vi "VCA_S.vi"(6 "EG":fxp<+,8,0>=0.99609375, 8 "Amount":fxp<+,8,0>=0.99609375, 9 "Sample In":fxp<+/-,8,8>) -> (1 "Sample Out":fxp<+/-,8,8>)   [LabVIEW 2015]
doc: "Includes two steps of amplitude control, adding flexibility to more complex signal generator designs.\n\nThe latency of this VI is 14 cycles."
uses:
  <vilib>/rvi/FXPMathLib/FxpMul/XNode/nifxpmath_Multiplier.xnode
  <vilib>/rvi/FXPMathLib/sim/FxpSim.dll
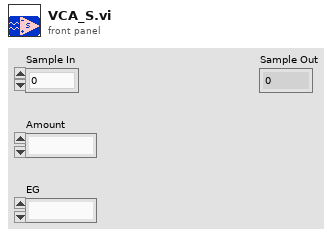
[diagram p1: front panel]
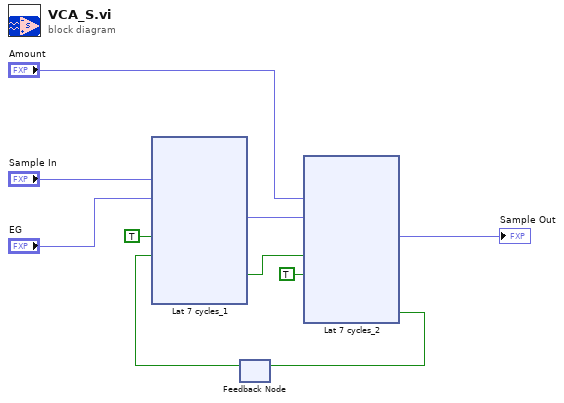
[diagram p0: block diagram]
diagram:
  n1 = feedback #1() -> (w3:bool)  [unwired: 1 in]
  n2 = xnode "Lat 7 cycles_1"("x"="Sample In", "y"="EG", "input valid"=TRUE, "ready for output (T)"=w3) -> ("x*y"=w6:fxp<+/-,8,8>, "output valid"=w2:bool)  [unwired: 1 out]
  n3 = xnode "Lat 7 cycles_2"("x"="Amount", "y"=w6, "input valid"=w2, "ready for output (T)"=TRUE) -> ("x*y"=→"Sample Out":fxp<+/-,8,8>, "ready for input"=w4:bool)  [unwired: 1 out]
  n4 = feedback-in #1(w4) -> ()
